vi "Init.vi"(8 "error in (no error)":errorcluster, 11 "Data":variant) -> (0 "error out":errorcluster)   [LabVIEW 2026, in "Display.lvlib"]
doc: "For named purposes"
uses:
  Display.lvlib
  Private Control/Queue Element.ctl
  Private Control/Module Action.ctl
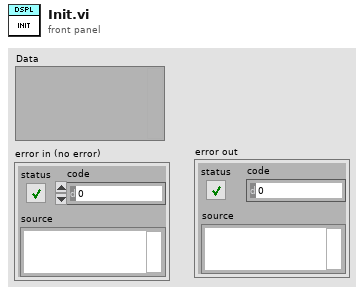
[diagram p1: front panel]
types:
  T1 = typedef "Display.lvlib/Queue Element.ctl" = cluster{"Module Action":T2, "Data":variant}
  T2 = typedef "Display.lvlib/Module Action.ctl" = enum16{"Init", "Error", "Exit"}
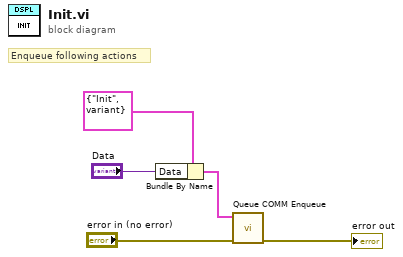
[diagram p0: block diagram]
diagram:
  # "Enqueue following actions"
  n1 = Bundle By Name(cluster=T1 {"Module Action"=enum."Init", "Data"=variant} ("element"), "Data"="Data") -> (w3:T1)
  n2 = call "Queue COMM Enqueue.vi"("error in (no error)"="error in (no error)", "element"=w3) -> ("error out"=→"error out":errorcluster)  [unwired: 9 in]
